vi "UI_WindowFrame3.vi"   [LabVIEW 2020]
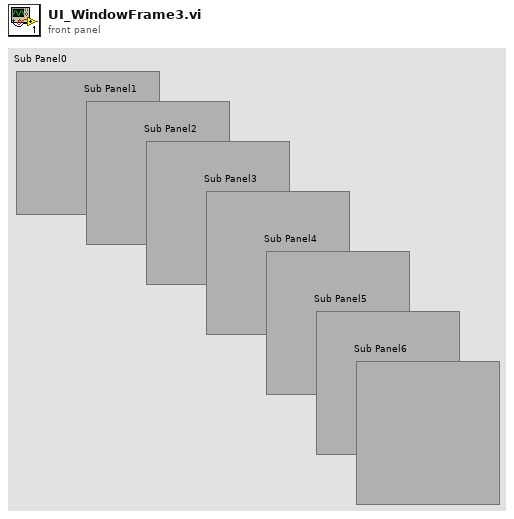
[diagram p1: front panel]
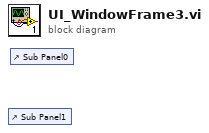
[diagram p0: block diagram]
diagram:
  n1 = control-ref of="Sub Panel1"() -> ()  [unwired: 1 out]
  n2 = control-ref of="Sub Panel0"() -> ()  [unwired: 1 out]
